vi "SQL_test_template_select.vi"() -> (0 "error out":errorcluster, 3 "表格控件":string[][](table))   [LabVIEW 2014]
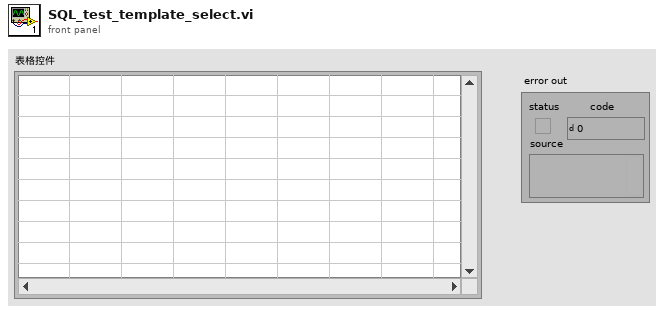
[diagram p1: front panel]
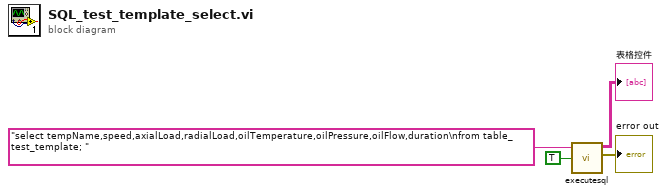
[diagram p0: block diagram]
diagram:
  n1 = call "executesql.vi"("Return Data (T)"=TRUE, "Command Text"="select tempName,speed,axialLoad,radialLoad,oilTemperature,oilPressure,oilFlow,duration\nfrom table_test_template; ") -> ("error out"=→"error out":errorcluster, "Data"=→"表格控件":string[][])  [unwired: 5 in]
